vi "IntakeFwdRevControl.vi"(5 "Intake Reverse":bool, 6 "Intake Forward":bool, 7 "IntakeMaxSpeed":dbl=1.0) -> (0 "IntakeOpen":bool, 1 "IntakeExtend":bool, 2 "ClawClose":bool, 3 "Intake Speed":dbl)   [LabVIEW 2017]
uses:
  TypeDefs/IntakeState.ctl
  ArgosLib/ArgosLib.lvlib
panel:
  in  "IntakeCloseDelay (s)":dbl=0.125
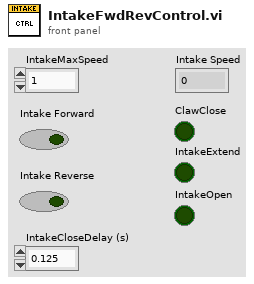
[diagram p1: front panel]
types:
  T1 = typedef "IntakeState.ctl" = enum16{"Stop", "Forward", "Reverse"}
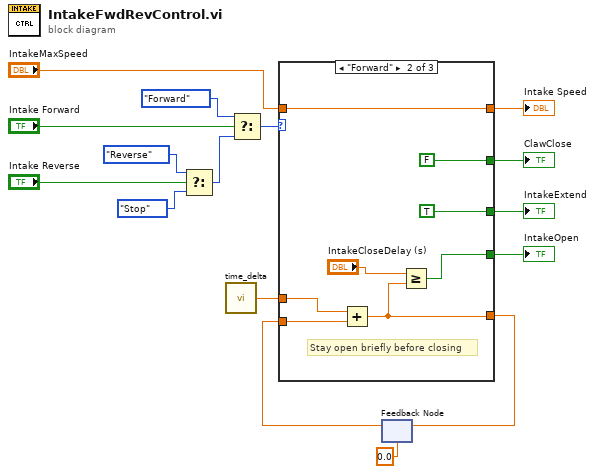
[diagram p0: block diagram]
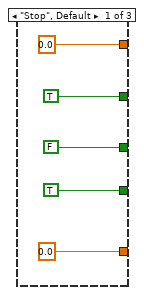
[diagram p2: hidden frame]
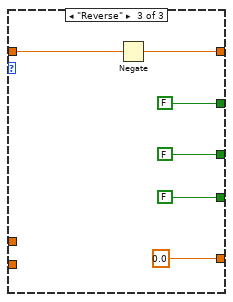
[diagram p3: hidden frame]
diagram:
  n1 = Select(t=IntakeState."Reverse", s="Intake Reverse", f=IntakeState."Stop" ("IntakeState")) -> (s? t:f=w14:T1)
  n2 = call "time_delta.vi"() -> ("dt (s)"=w1:dbl)  [unwired: 1 in]
  n3 = Select(t=IntakeState."Forward", s="Intake Forward", f=w14) -> (s? t:f=w10:T1)
  n4 = feedback #1(0.0) -> (w3:dbl)
  n5 = case shown="\"Forward\"" w10 {
    tunnel: [0.0 ("Intake Speed") w29 w34] -> w9
    tunnel: [TRUE ("ClawClose") FALSE ("ClawClose") FALSE ("ClawClose")] -> w8
    tunnel: [FALSE ("IntakeExtend") TRUE ("IntakeExtend") FALSE ("IntakeExtend")] -> w7
    tunnel: [TRUE ("IntakeOpen") w22 FALSE ("IntakeOpen")] -> w6
    tunnel: "IntakeMaxSpeed" -> [_ w29 w35]
    tunnel: [0.0 w23 0.0] -> w4
    tunnel: w3 -> [_ w26 _]
    tunnel: w1 -> [_ w25 _]
    frame "Stop", Default {
    }
    frame "Forward" {
      # "Stay open briefly before closing"
      n6 = Add(x=w25, y=w26) -> (x+y=w23:dbl)
      n7 = Greater Or Equal?(x="IntakeCloseDelay (s)", y=w23) -> (x >= y?=w22:bool)
    }
    frame "Reverse" {
      n8 = Negate(x=w35) -> (-x=w34:dbl)
    }
  }
  "ClawClose" <- w8
  "Intake Speed" <- w9
  "IntakeExtend" <- w7
  "IntakeOpen" <- w6
  n9 = feedback-in #1(w4) -> ()
